vi "Publish FC2 ILC Outputs.vi"(8 "error in (no error)":errorcluster, 11 "Model in":refnum<class "Model.lvclass">) -> (0 "error out":errorcluster, 3 "Model out":refnum<class "Model.lvclass">)   [LabVIEW 2015, in "Model.lvclass"]
uses:
  Model.lvclass
  Model.lvclass/Model.ctl
  <userlib>/Common/ILC/ILC/ILC.lvclass/ILC.ctl
  UserEvents/UserEvents.lvclass/UserEvents.ctl
  UserEvents/UserEvents.lvclass
  <userlib>/Common/ILC/ILC/ILC.lvclass
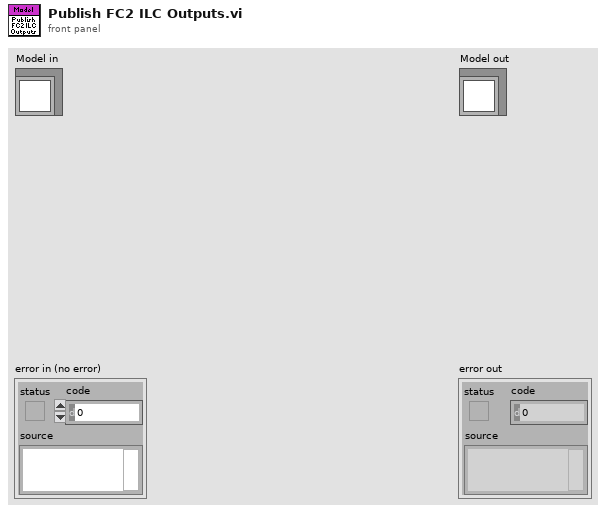
[diagram p1: front panel]
types:
  T1 = typedef "ILCCommon.lvlib/ILCTypedefs.lvlib/Outputs.ctl" = cluster{"Step & Direction":i16, "Blower RPM":u8, "PWM (SSR)":u8, "Ch1":u16, "Ch2":u16, "Ch3":u16, "Ch4":u16}
  T2 = typedef "FAMT Typedefs.lvlib/Publish Data Events.ctl" = cluster{"State":refnum<user-event>, "ErrorCode":refnum<user-event>, "FC1 ILC Outputs":refnum<user-event>, "LogPath":refnum<user-event>, "FC1 ILC Inputs":refnum<user-event>, "Scan Progress":refnum<user-event>, "FC2 ILC Outputs":refnum<user-event>, "FC2 ILC Inputs":refnum<user-event>}
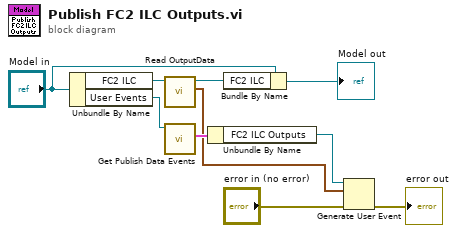
[diagram p0: block diagram]
diagram:
  n1 = Unbundle By Name("Model in") -> ("FC2 ILC"=w9:refnum<class "ILC.lvclass">, "User Events"=w3:refnum<class "UserEvents.lvclass">)
  n2 = call <userlib>:"Read OutputData.vi"("ILC in"=w9) -> ("OutputData"=w2:T1, "ILC out"=w6:refnum<class "ILC.lvclass">)  [unwired: 9 in]
  n3 = call "Get Publish Data Events.vi"("UserEvents in"=w3) -> ("Publish Data Events"=w10:T2)  [unwired: 9 in, 1 out]
  n4 = Unbundle By Name(w10) -> ("FC2 ILC Outputs"=w8:refnum<user-event>)
  n5 = Bundle By Name(cluster="Model in", "FC2 ILC"=w6) -> (→"Model out":refnum<class "Model.lvclass">)
  n6 = Generate User Event(user event=w8, event data cluster=w2, error in="error in (no error)") -> (error out=→"error out":errorcluster)  [unwired: 1 in, 1 out]
